vi "ErrorHandling.Main.vi"() -> ()   [LabVIEW 2016, in "ErrorHandling.lvclass"]
doc: "The ErrorHandlings Main VI keeps the ErrorHandling Object. The ErrorHandler Object can't be saved in the Object Handler (Package Resource Control) since ErrorHandling is initiated before the ObjectHandler is initiated.\n\nAndreas Elmiger, 04.01.2017"
uses:
  ErrorHandling.lvclass
  Package Libraries/Message Queue/private/MessageQueue.MessageTypeDef.ctl
  ErrorHandling.lvclass/ErrorHandling.ctl
  Package ResourceControl/ObjectHandler/ObjectHandler.GetObjectWType.ctl
  Package Libraries/StringFunctions/StringFunctions_ReplaceAllBlindSigns.vi
  <vilib>/Utility/error.llb/Clear Errors.vi
  <vilib>/dlg_ctls.llb/Space Constant.vi
  <vilib>/Utility/error.llb/Trim Whitespace.vi
  <vilib>/Utility/error.llb/Search and Replace Pattern.vi
  Package Libraries/TimingFunctions/TimingFunctions_getUtcTimestamp.vi
  ErrorHandling.addLastErrorToFile.vi
  Package ResourceControl/ObjectHandler/ObjectHandler.lvclass
panel:
  in  "ErrorList":i32(listbox)
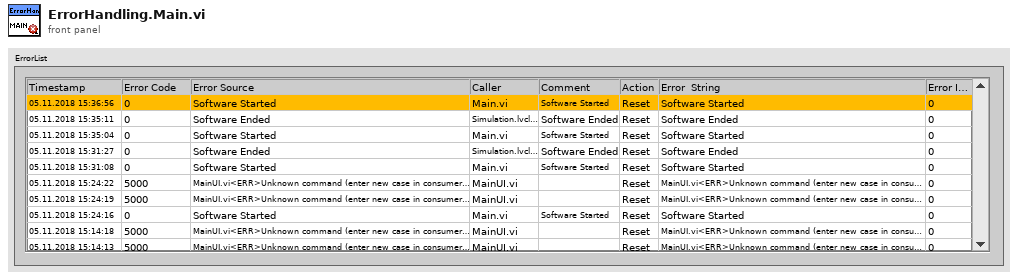
[diagram p1: front panel]
types:
  T1 = typedef "MessageQueue.MessageTypeDef.ctl" = cluster{"Message":string, "Data":variant}
  T2 = typedef "ObjectHandler.lvclass/ObjectHandler.GetObjectWType.ctl" = cluster{"Name":string, "Caller":string}
  T3 = typedef "ErrorHandling.lvclass/ErrorHandling.OccurredErrorDataStruct.ctl" = cluster{"Error":errorcluster, "Caller":string, "Comment":string, "Timestamp":timestamp, "Stopped":bool, "ErrorCusterString":string, "ErrorIndex":u64}
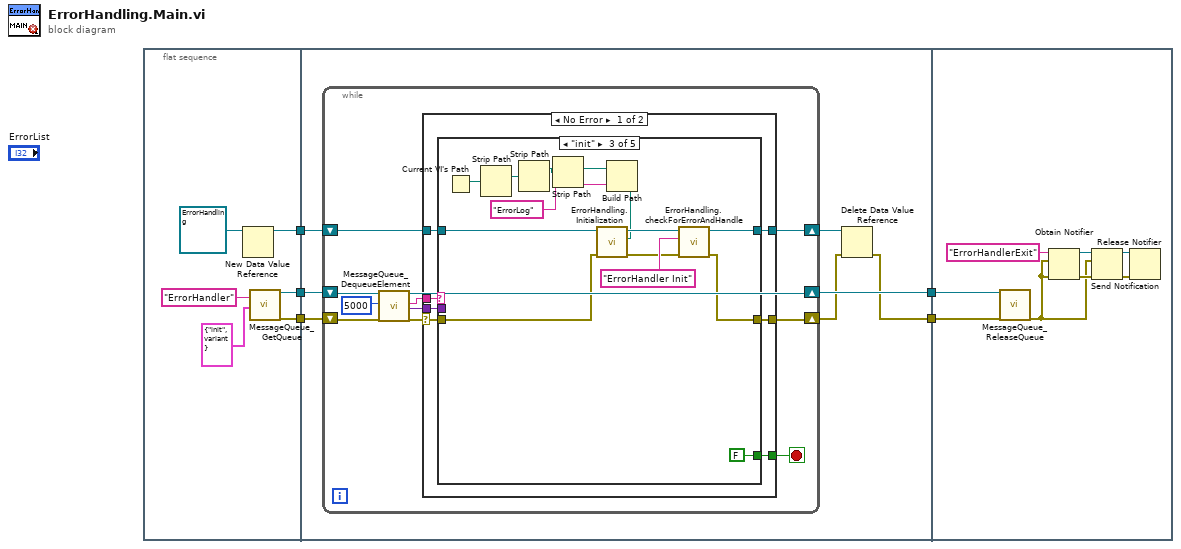
[diagram p0: block diagram]
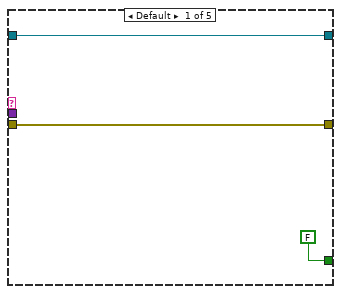
[diagram p2: hidden frame]
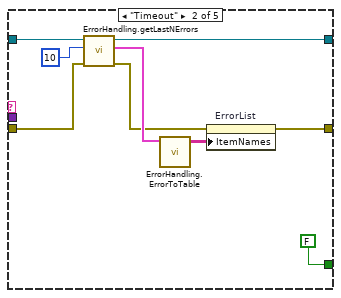
[diagram p3: hidden frame]
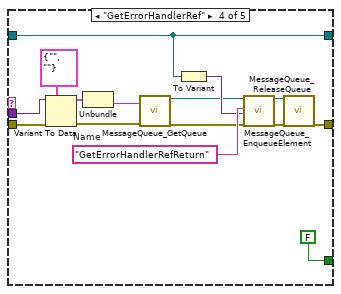
[diagram p4: hidden frame]
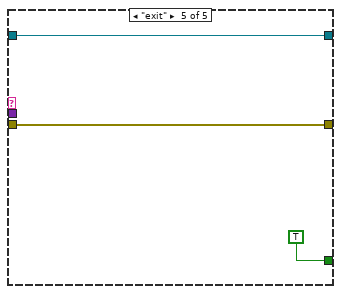
[diagram p5: hidden frame]
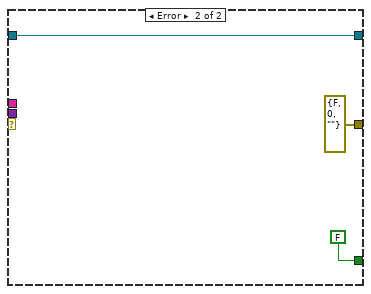
[diagram p6: hidden frame]
diagram:
  n1 = flat-sequence {
    tunnel: [w6] -> w5
    tunnel: [w10] -> w4
    tunnel: [w9] -> w3
    tunnel: w5 -> [w16]
    tunnel: w4 -> [w18]
    tunnel: w3 -> [w17]
    tunnel: [w12] -> w2
    tunnel: [w15] -> w1
    tunnel: w2 -> [w91]
    tunnel: w1 -> [w90]
    frame #0 {
      n2 = New Data Value Reference(data value=refnum<class "ErrorHandling.lvclass"> refnum ("ErrorHandling.lvclass")) -> (data value reference=w6:refnum<data-value>)  [unwired: 1 in, 1 out]
      n3 = call "MessageQueue_GetQueue.vi"("Name"="ErrorHandler", "OptionalInitValue"=T1 {"Message"="init", "Data"=variant}) -> ("QueueOut"=w10:refnum<queue>, "ErrorOut"=w9:errorcluster)  [unwired: 15 in, 1 out]
    }
    frame #1 {
      n4 = while {
        shift-right: [w23] -> w14
        shift-left: w16 -> [w24]
        shift-right: [w22] -> w13
        shift-left: w17 -> [w29]
        shift-right: [w20] -> w15
        shift-left: w18 -> [w28]
        stop <- w21 stop-if-true
        n5 = call "MessageQueue_DequeueElement.vi"("QueueIn"=w28, "Timeout"=5000, "ErrorIn"=w29) -> ("QueueOut"=w20:refnum<queue>, "Message"=w26:string, "Data"=w25:variant, "ErrorOut"=w27:errorcluster)  [unwired: 12 in, 1 out]
        n6 = case shown="No Error" w27 {
          selector: w27 -> [w34 _]
          tunnel: w26 -> [w36 _]
          tunnel: w25 -> [w35 _]
          tunnel: w24 -> [w33 w83]
          tunnel: [w32 w83] -> w23
          tunnel: [w31 errorcluster {"status"=FALSE, "code"=0, "source"=""} ("error out")] -> w22
          tunnel: [w30 FALSE] -> w21
          frame No Error {
            n7 = case shown="\"init\"" w36 {
              tunnel: w35 -> [_ _ _ w65 _]
              tunnel: w34 -> [w38 w47 w51 w68 w78]
              tunnel: w33 -> [w39 w45 w61 w66 w79]
              tunnel: [w39 w44 w58 w66 w79] -> w32
              tunnel: [w38 w40 w57 w67 w78] -> w31
              tunnel: [FALSE FALSE FALSE FALSE TRUE] -> w30
              frame Default {
              }
              frame "Timeout" {
                n8 = call "ErrorHandling.getLastNErrors.vi"("error in (no error)"=w47, "N"=u32 10, "ErrorHandling in"=w45) -> ("error out"=w41:errorcluster, "Errors"=w43:T3[], "ErrorHandling out"=w44:refnum<data-value>)  [unwired: 6 in]
                n9 = call "ErrorHandling.ErrorToTable.vi"("Errors"=w43) -> ("Item Names"=w42:string[][])  [unwired: 10 in]
                n10 = property on="ErrorList" class="MCListbox (strict)"(error in=w41, "ItemNames"=w42) -> (error out=w40:errorcluster)  [unwired: 1 in, 1 out]
              }
              frame "init" {
                n11 = Current VI's Path() -> (path=w49:path)
                n12 = Strip Path(path=w49) -> (stripped path=w56:path)  [unwired: 1 out]
                n13 = Strip Path(path=w56) -> (stripped path=w53:path)  [unwired: 1 out]
                n14 = Strip Path(path=w53) -> (stripped path=w50:path)  [unwired: 1 out]
                n15 = Build Path(base path=w50, name or relative path="ErrorLog") -> (appended path=w52:path)
                n16 = call "ErrorHandling.Initialization.vi"("error in"=w51, "ErrorBasePath"=w52, "ErrorHandling(optional)"=w61) -> ("error out"=w54:errorcluster, "ErrorHandling out"=w59:refnum<data-value>)  [unwired: 7 in]
                n17 = call "ErrorHandling.checkForErrorAndHandle.vi"("error in (no error)"=w54, "Comment"="ErrorHandler Init" ("Comment(optional)"), "ErrorHandling in"=w59) -> ("error out"=w57:errorcluster, "ErrorHandling out"=w58:refnum<data-value>)  [unwired: 6 in, 1 out]
              }
              frame "GetErrorHandlerRef" {
                w77 = "GetErrorHandlerRefReturn"  # Name
                n18 = Variant To Data(error in=w68, type=T2 {"Name"="", "Caller"=""} ("GetRefInput"), Variant=w65) -> (data=w70:T2, error out=w72:errorcluster)
                n19 = Unbundle(w70) -> ("Caller"=w71:string)  [unwired: 1 out]
                n20 = call "MessageQueue_GetQueue.vi"("Name"=w71, "ErrorIn"=w72) -> ("QueueOut"=w73:refnum<queue>, "ErrorOut"=w64:errorcluster)  [unwired: 15 in, 1 out]
                n21 = To Variant(anything=w66) -> (Variant=w76:variant)
                n22 = call "MessageQueue_EnqueueElement.vi"("QueueIn"=w73, "Message"=w77, "Data"=w76, "ErrorIn"=w64) -> ("QueueOut"=w75:refnum<queue>, "ErrorOut"=w74:errorcluster)  [unwired: 14 in]
                n23 = call "MessageQueue_ReleaseQueue.vi"("QueueIn"=w75, "ErrorIn"=w74) -> ("ErrorOut"=w67:errorcluster)  [unwired: 15 in, 2 out]
              }
              frame "exit" {
              }
            }
          }
          frame Error {
          }
        }
      }
      n24 = Delete Data Value Reference(data value reference=w14, error in=w13) -> (error out=w12:errorcluster)  [unwired: 1 out]
    }
    frame #2 {
      n25 = call "MessageQueue_ReleaseQueue.vi"("QueueIn"=w90, "ErrorIn"=w91) -> ("ErrorOut"=w86:errorcluster)  [unwired: 15 in, 2 out]
      n26 = Obtain Notifier(name (unnamed)="ErrorHandlerExit", notification data type=w86, error in (no error)=w86) -> (notifier out=w87:refnum<notifier>, error out=w88:errorcluster)  [unwired: 1 in, 1 out]
      n27 = Send Notification(notification=w86, notifier=w87, error in (no error)=w88) -> (notifier out=w84:refnum<notifier>, error out=w85:errorcluster)
      n28 = Release Notifier(notifier=w84, error in (no error)=w85) -> ()  [unwired: 1 in, 3 out]
    }
  }
